vi "ComputeDesiredState.vi"(11 "Robot Action Array":T1) -> ()   [LabVIEW 2019]
uses:
  Controls/Robot Actions Array.ctl
  Controls/Robot Actions.ctl
  Controls/Robot State.ctl
  Controls/Robot Pivot Motion Commands.ctl
  Controls/Pivot Motor Commands.ctl
  Controls/Robot Drive Mode.ctl
  Controls/Enable Actions.ctl
  Controls/Lift System Actions.ctl
  Controls/Spinner Actions.ctl
  Controls/Ball System Actions.ctl
  Controls/DriveJoystickData.ctl
  Global Variables/Trajectory Enabled.vi
  <vilib>/Rock Robotics/Network Tables/NT Write Number.vi
  Global Variables/Robot State.vi
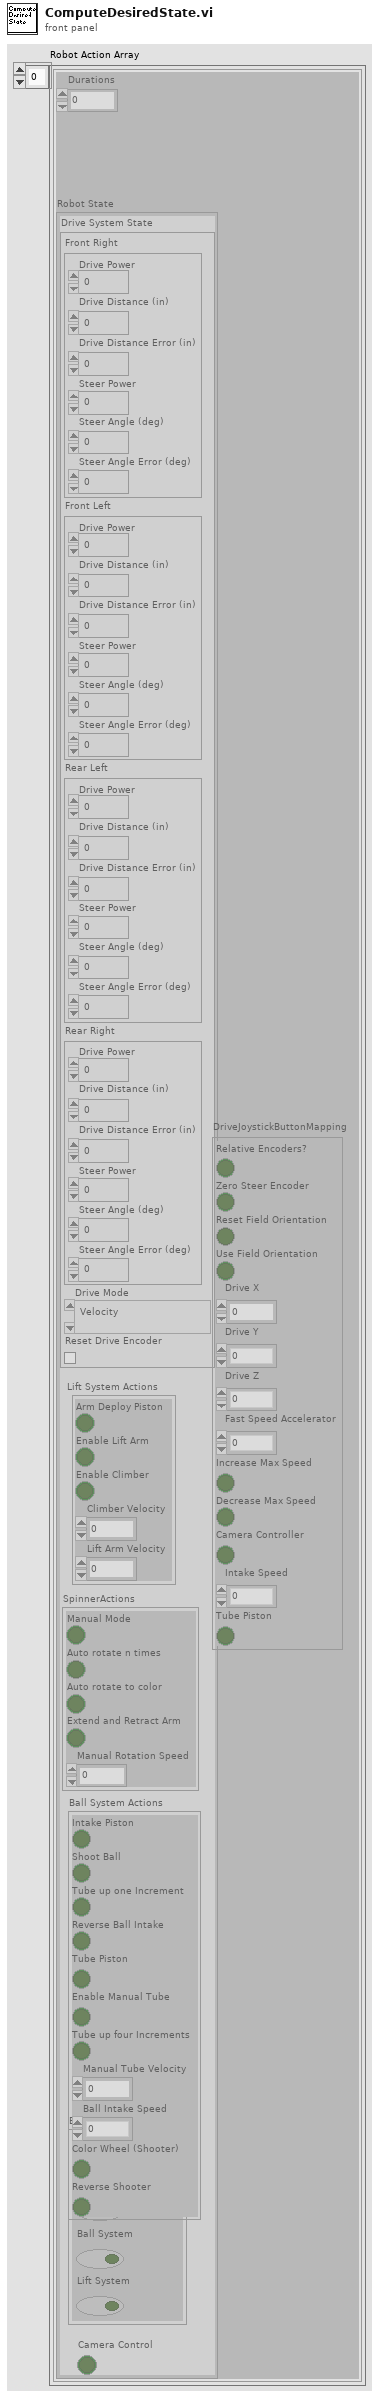
[diagram p1: front panel]
types:
  T1 = typedef "Robot Actions Array.ctl" = T2[]
  T2 = typedef "Robot Actions.ctl" = cluster{"Durations":dbl, "Robot State":T3, "DriveJoystickButtonMapping":T11}
  T3 = typedef "Robot State.ctl" = cluster{"Drive System State":T4, "Enable Actions":T7, "Lift System Actions":T8, "SpinnerActions":T9, "Ball System Actions":T10, "Camera Control":bool}
  T4 = typedef "Robot Pivot Motion Commands.ctl" = cluster{"Front Right":T5, "Front Left":T5, "Rear Left":T5, "Rear Right":T5, "Drive Mode":T6, "Reset Drive Encoder":bool}
  T5 = typedef "Pivot Motor Commands.ctl" = cluster{"Drive Power":dbl, "Drive Distance (in)":dbl, "Drive Distance Error (in)":dbl, "Steer Power":dbl, "Steer Angle (deg)":dbl, "Steer Angle Error (deg)":dbl}
  T6 = typedef "Robot Drive Mode.ctl" = enum16{"Velocity", "Distance"}
  T7 = typedef "Enable Actions.ctl" = cluster{"Manual Swerve Drive":bool, "Color System":bool, "Ball System":bool, "Lift System":bool}
  T8 = typedef "Lift System Actions.ctl" = cluster{"Arm Deploy Piston":bool, "Enable Lift Arm":bool, "Enable Climber":bool, "Climber Velocity":dbl, "Lift Arm Velocity":dbl}
  T9 = typedef "Spinner Actions.ctl" = cluster{"Manual Mode ":bool, "Auto rotate n times":bool, "Auto rotate to color\t":bool, "Extend and Retract Arm\t":bool, "Manual Rotation Speed":dbl}
  T10 = typedef "Ball System Actions.ctl" = cluster{"Intake Piston ":bool, "Shoot Ball":bool, "Tube up one Increment\t":bool, "Reverse Ball Intake":bool, "Tube Piston":bool, "Enable Manual Tube":bool, "Tube up four Increments":bool, "Manual Tube Velocity":dbl, "Ball Intake Speed":dbl, "Color Wheel (Shooter)":bool, "Reverse Shooter":bool}
  T11 = typedef "DriveJoystickData.ctl" = cluster{"Relative Encoders?":bool, "Zero Steer Encoder":bool, "Reset Field Orientation":bool, "Use Field Orientation":bool, "Drive X":dbl, "Drive Y":dbl, "Drive Z":dbl, "Fast Speed Accelerator":dbl, "Increase Max Speed":bool, "Decrease Max Speed":bool, "Camera Controller":bool, "Intake Speed":dbl, "Tube Piston":bool}
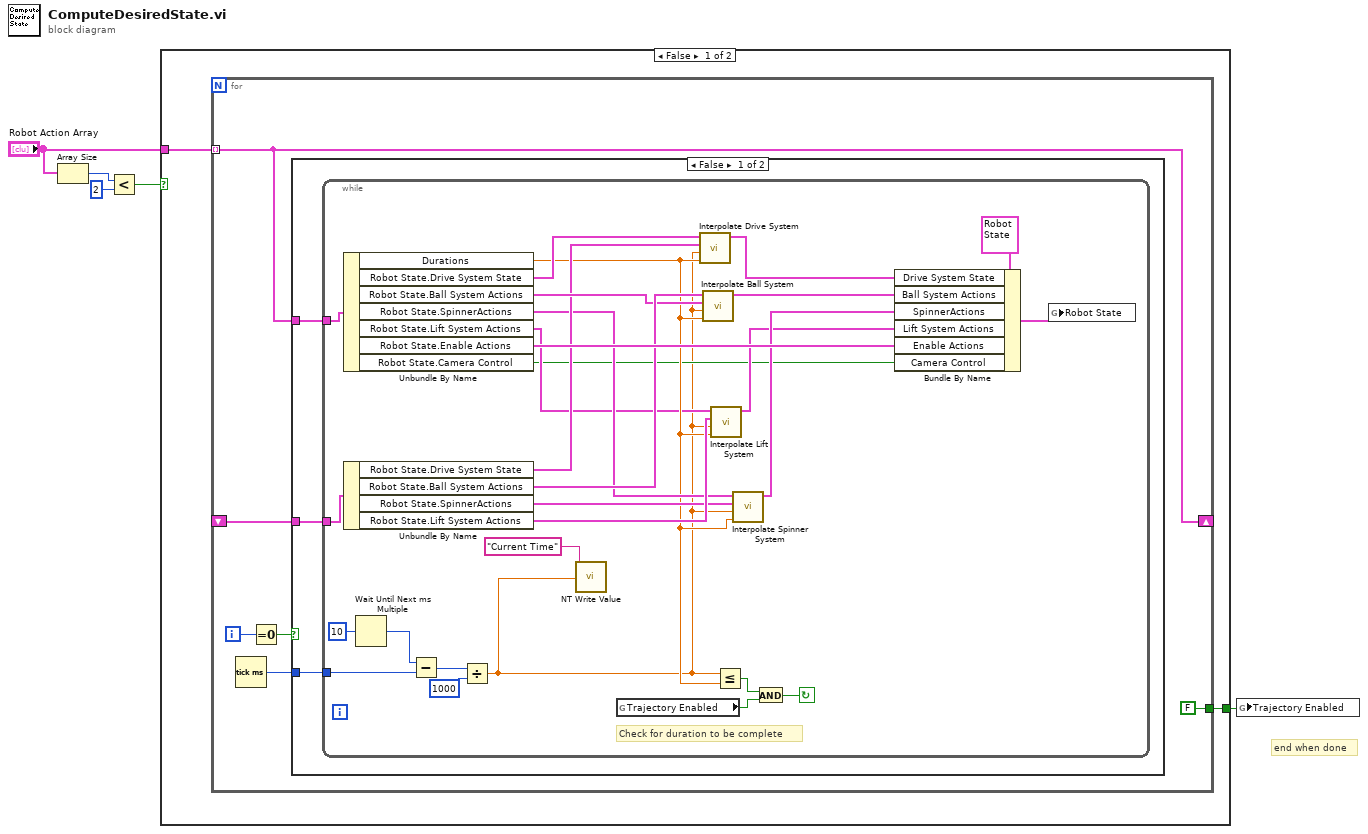
[diagram p0: block diagram]
diagram:
  # "end when done"
  n1 = Array Size(array="Robot Action Array") -> (size(s)=w3:i32)
  n2 = Less?(x=w3, y=2) -> (x < y?=w1:bool)
  n3 = case shown="False" w1 {
    tunnel: [w7 _] -> w5
    tunnel: "Robot Action Array" -> [w6 _]
    frame False {
      n4 = for {
        tunnel: w6 -> [w10] mode=indexing
        shift-right: [w10] -> _
        shift-left: _ -> [w11]
        tunnel: [FALSE ("Trajectory Enabled")] -> w7
        i -> [w13]
        n5 = Tick Count (ms)() -> (millisecond timer value=w9:u32)
        n6 = Equal To 0?(x=w13) -> (x = 0?=w12:bool)
        n7 = case shown="False" w12 {
          tunnel: w11 -> [w15 _]
          tunnel: w10 -> [w16 _]
          tunnel: w9 -> [w14 _]
          frame False {
            n8 = while {
              tunnel: w16 -> [w44]
              tunnel: w15 -> [w45]
              tunnel: w14 -> [w38]
              stop <- w33 continue-if-true
              # "Check for duration to be complete"
              n9 = Unbundle By Name(w44) -> ("Durations"=w22:dbl, "Robot State.Drive System State"=w28:T4, "Robot State.Ball System Actions"=w30:T10, "Robot State.SpinnerActions"=w25:T9, "Robot State.Lift System Actions"=w21:T8, "Robot State.Enable Actions"=w41:T7, "Robot State.Camera Control"=w19:bool)
              n10 = Unbundle By Name(w45) -> ("Robot State.Drive System State"=w29:T4, "Robot State.Ball System Actions"=w31:T10, "Robot State.SpinnerActions"=w24:T9, "Robot State.Lift System Actions"=w26:T8)
              n11 = Wait Until Next ms Multiple(millisecond multiple=u32 10) -> (millisecond timer value=w39:u32)
              n12 = Subtract(x=w39, y=w38) -> (x-y=w37:u32)
              n13 = Divide(x=w37, y=u32 1000) -> (x/y=w18:dbl)
              n14 = call-poly <vilib>:"NT Write Value.vi"("Numeric"=w18, "Name"="Current Time") -> ()  [unwired: 9 in, 1 out]
              n15 = global read "Trajectory Enabled.vi" "Trajectory Enabled"() -> (w34:bool)
              n16 = call "Interpolate Drive System.vi"("Duration"=w22, "Current Time"=w18, "Start Robot Commands"=w29, "End Robot Commands"=w28) -> ("Current Robot Commands"=w27:T4)  [unwired: 7 in]
              n17 = call "Interpolate Ball System.vi"("Duration"=w22, "Current Time"=w18, "End Ball System Actions"=w30, "Start Ball System Actions"=w31) -> ("Ball System Actions"=w40:T10)  [unwired: 7 in]
              n18 = call "Interpolate Lift System.vi"("Duration"=w22, "Current Time"=w18, "End Lift System Actions"=w26, "Start Lift System Actions"=w21) -> ("Current Lift System Actions"=w20:T8)  [unwired: 7 in]
              n19 = Less Or Equal?(x=w18, y=w22) -> (x <= y?=w35:bool)
              n20 = call "Interpolate Spinner System.vi"("Duration"=w22, "Current Time"=w18, "End SpinnerActions"=w24, "Start SpinnerActions"=w25) -> ("Current SpinnerActions"=w23:T9)  [unwired: 7 in]
              n21 = And(x=w35, y=w34) -> (x .and. y?=w33:bool)
              n22 = Bundle By Name(cluster=T3 {"Drive System State"={"Front Right"={"Drive Power"=0.0, "Drive Distance (in)"=0.0, "Drive Distance Error (in)"=0.0, "Steer Power"=0.0, "Steer Angle (deg)"=0.0, "Steer Angle Error (deg)"=0.0}, "Front Left"={"Drive Power"=0.0, "Drive Distance (in)"=0.0, "Drive Distance Error (in)"=0.0, "Steer Power"=0.0, "Steer Angle (deg)"=0.0, "Steer Angle Error (deg)"=0.0}, "Rear Left"={"Drive Power"=0.0, "Drive Distance (in)"=0.0, "Drive Distance Error (in)"=0.0, "Steer Power"=0.0, "Steer Angle (deg)"=0.0, "Steer Angle Error (deg)"=0.0}, "Rear Right"={"Drive Power"=0.0, "Drive Distance (in)"=0.0, "Drive Distance Error (in)"=0.0, "Steer Power"=0.0, "Steer Angle (deg)"=0.0, "Steer Angle Error (deg)"=0.0}, "Drive Mode"=enum."Velocity", "Reset Drive Encoder"=FALSE}, "Enable Actions"={"Manual Swerve Drive"=FALSE, "Color System"=FALSE, "Ball System"=FALSE, "Lift System"=FALSE}, "Lift System Actions"={"Arm Deploy Piston"=FALSE, "Enable Lift Arm"=FALSE, "Enable Climber"=FALSE, "Climber Velocity"=0.0, "Lift Arm Velocity"=0.0}, "SpinnerActions"={"Manual Mode "=FALSE, "Auto rotate n times"=FALSE, "Auto rotate to color\t"=FALSE, "Extend and Retract Arm\t"=FALSE, "Manual Rotation Speed"=0.0}, "Ball System Actions"={"Intake Piston "=FALSE, "Shoot Ball"=FALSE, "Tube up one Increment\t"=FALSE, "Reverse Ball Intake"=FALSE, "Tube Piston"=FALSE, "Enable Manual Tube"=FALSE, "Tube up four Increments"=FALSE, "Manual Tube Velocity"=0.0, "Ball Intake Speed"=0.0, "Color Wheel (Shooter)"=FALSE, "Reverse Shooter"=FALSE}, "Camera Control"=FALSE} ("Robot State"), "Drive System State"=w27, "Ball System Actions"=w40, "SpinnerActions"=w23, "Lift System Actions"=w20, "Enable Actions"=w41, "Camera Control"=w19) -> (w42:T3)
              n23 = global write "Robot State.vi" "Robot State"(w42) -> ()
            }
          }
          frame True {
            # "Ignore the first time through the loop because it is the starting point for the trajectory."
          }
        }
      }
    }
    frame True {
      # "Do nothing.  not enough points in trajectory"
    }
  }
  n24 = global write "Trajectory Enabled.vi" "Trajectory Enabled"(w5) -> ()
